vi "ramper_up_auton.vi"(8 "Rate":dbl, 9 "Target Setpoint":dbl) -> (0 "Current Setpoint":dbl, 1 "Ramping":bool)   [LabVIEW 2011]
panel:
  out "crement":dbl
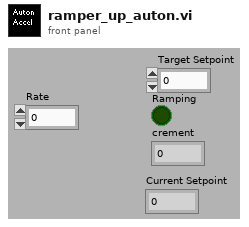
[diagram p1: front panel]
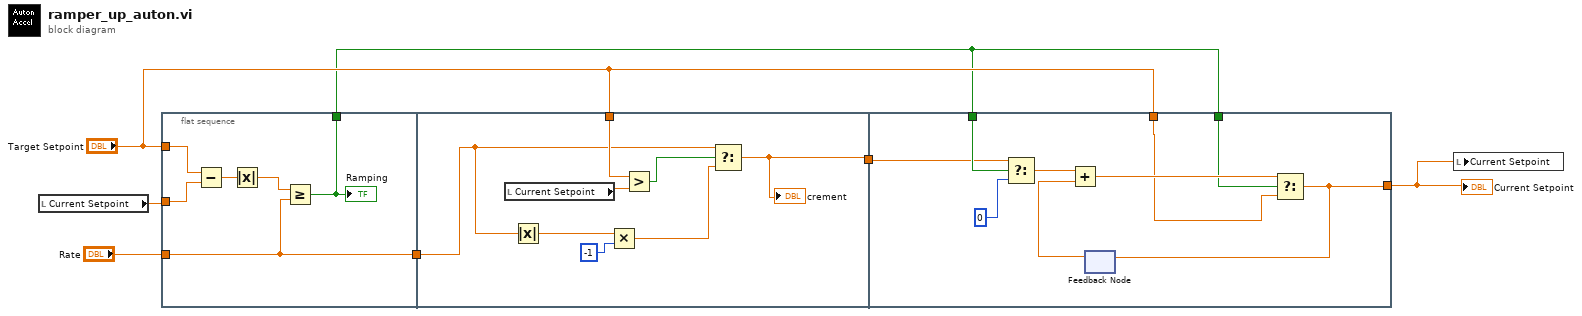
[diagram p0: block diagram]
diagram:
  n1 = local read "Current Setpoint"() -> (w1:dbl)
  n2 = flat-sequence {
    tunnel: "Target Setpoint" -> [w11]
    tunnel: w1 -> [w8]
    tunnel: "Rate" -> [w10]
    tunnel: [w10] -> w6
    tunnel: [w9] -> w3
    tunnel: "Target Setpoint" -> [w17]
    tunnel: w6 -> [w16]
    tunnel: [w15] -> w5
    tunnel: [w26] -> w2
    tunnel: w3 -> [w25]
    tunnel: w5 -> [w24]
    tunnel: "Target Setpoint" -> [w23]
    tunnel: w3 -> [w22]
    frame #0 {
      n3 = Subtract(x=w11, y=w8) -> (x-y=w12:dbl)
      n4 = Absolute Value(x=w12) -> (abs(x)=w13:dbl)
      n5 = Greater Or Equal?(x=w13, y=w10) -> (x >= y?=w9:bool)
      "Ramping" <- w9
    }
    frame #1 {
      n6 = local read "Current Setpoint"() -> (w14:dbl)
      n7 = Absolute Value(x=w16) -> (abs(x)=w20:dbl)
      n8 = Multiply(x=w20, y=-1) -> (x*y=w18:dbl)
      n9 = Greater?(x=w17, y=w14) -> (0:w21:bool)
      n10 = Select(t=w16, s=w21, f=w18) -> (s? t:f=w15:dbl)
      "crement" <- w15
    }
    frame #2 {
      n11 = Select(t=w24, s=w25, f=0) -> (s? t:f=w29:dbl)
      n12 = feedback #1() -> (w27:dbl)  [unwired: 1 out]
      n13 = Add(x=w29, y=w27) -> (x+y=w28:dbl)
      n14 = Select(t=w28, s=w22, f=w23) -> (s? t:f=w26:dbl)
      n15 = feedback-in #1(w26) -> ()
    }
  }
  n16 = local write "Current Setpoint"(w2) -> ()
  "Current Setpoint" <- w2
